vi "Program.vi"() -> ()   [LabVIEW 2018]
panel:
  in  "dados.txt":path
  in  "Error":bool
  in  "Notificacao Rapida":string
  in  "Tab Control":T1(tab)
  in  "DISCREPÂNCIA ACEITA(counts):":u16
  in  "Read-me":bool
  in  "VISUALIZA敲O DE DADOS":bool
  in  "PARAR EXECU敲O":bool
  in  "APAGAR DADOS ANTIGOS":bool
  out "EXECU敲O:":u16
  out "TABELA":string[][](table)
  out "Graph":cluster{"X":dbl[], "Y":dbl[]}[](graph) caption="XY Graph 2"
  in  "Reset":bool
  in  "Enviar Manualmente":bool
  in  "Envio Automático (Horas)":u8
  in  "Senha:":string
  in  "Porta SMTP":string
  in  "SMTP":string
  in  "Assunto:":string
  in  "Para":string[](array[string])
  in  "Email:":string
  in  "Enviar dados para Google Drive":bool
  in  "Enviar notificações por email":bool
  in  "Notificações":string
  in  "counts":dbl[](array[numeric])
  in  "size":i32
  in  "JSONe de Acesso ao Drive":path
  in  "tensao":dbl[](array[numeric])
  # "PAINEL DE CONTROLE"
  # "Gráfico de Counts vs Tensão"
  # "ENVIO DE NOTIFICA钦ES POR EMAIL"
  # "ENVIO AO GOOGLE DRIVE"
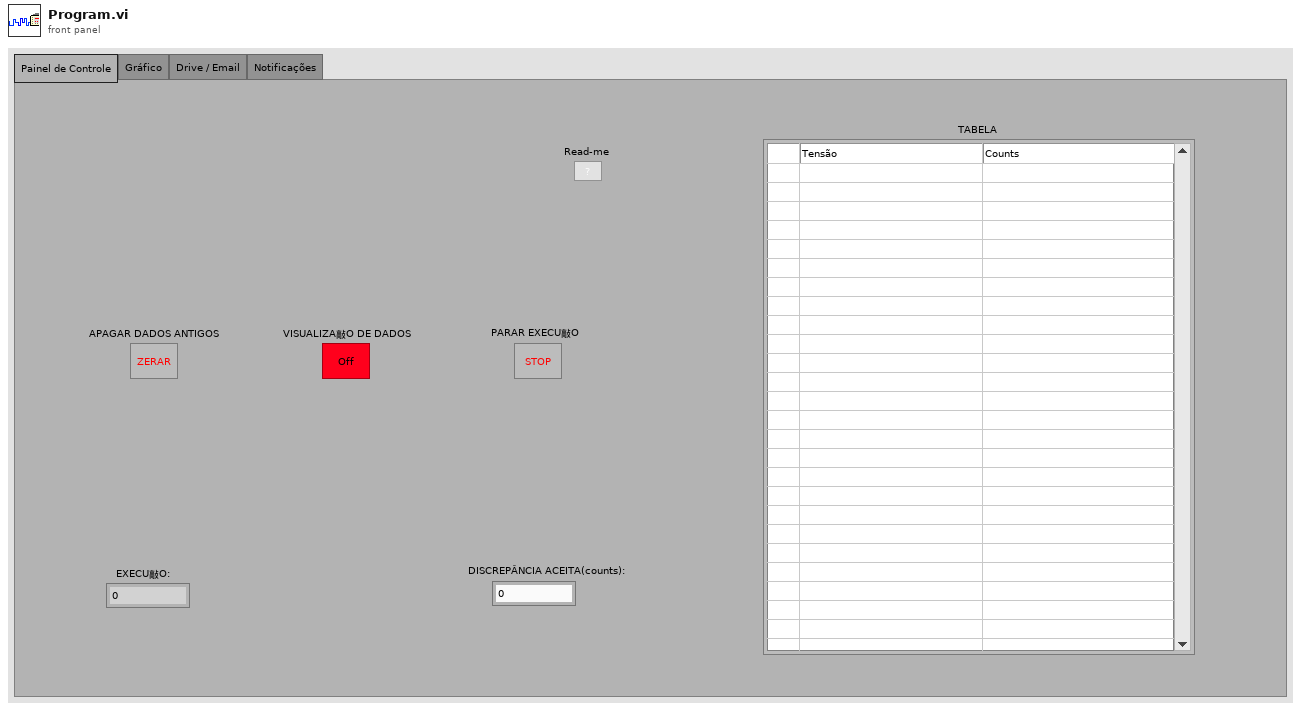
[diagram p1: front panel]
types:
  T1 = enum32{"Painel de Controle", "Gráfico", "Drive / Email", "Notificações"}
  T2 = enum32{"Invalid", "Standard", "Closed", "Hidden", "Minimized", "Maximized"}
  T3 = enum16{"open", "replace", "create", "open or create", "replace or create", "replace or create with confirmation"}
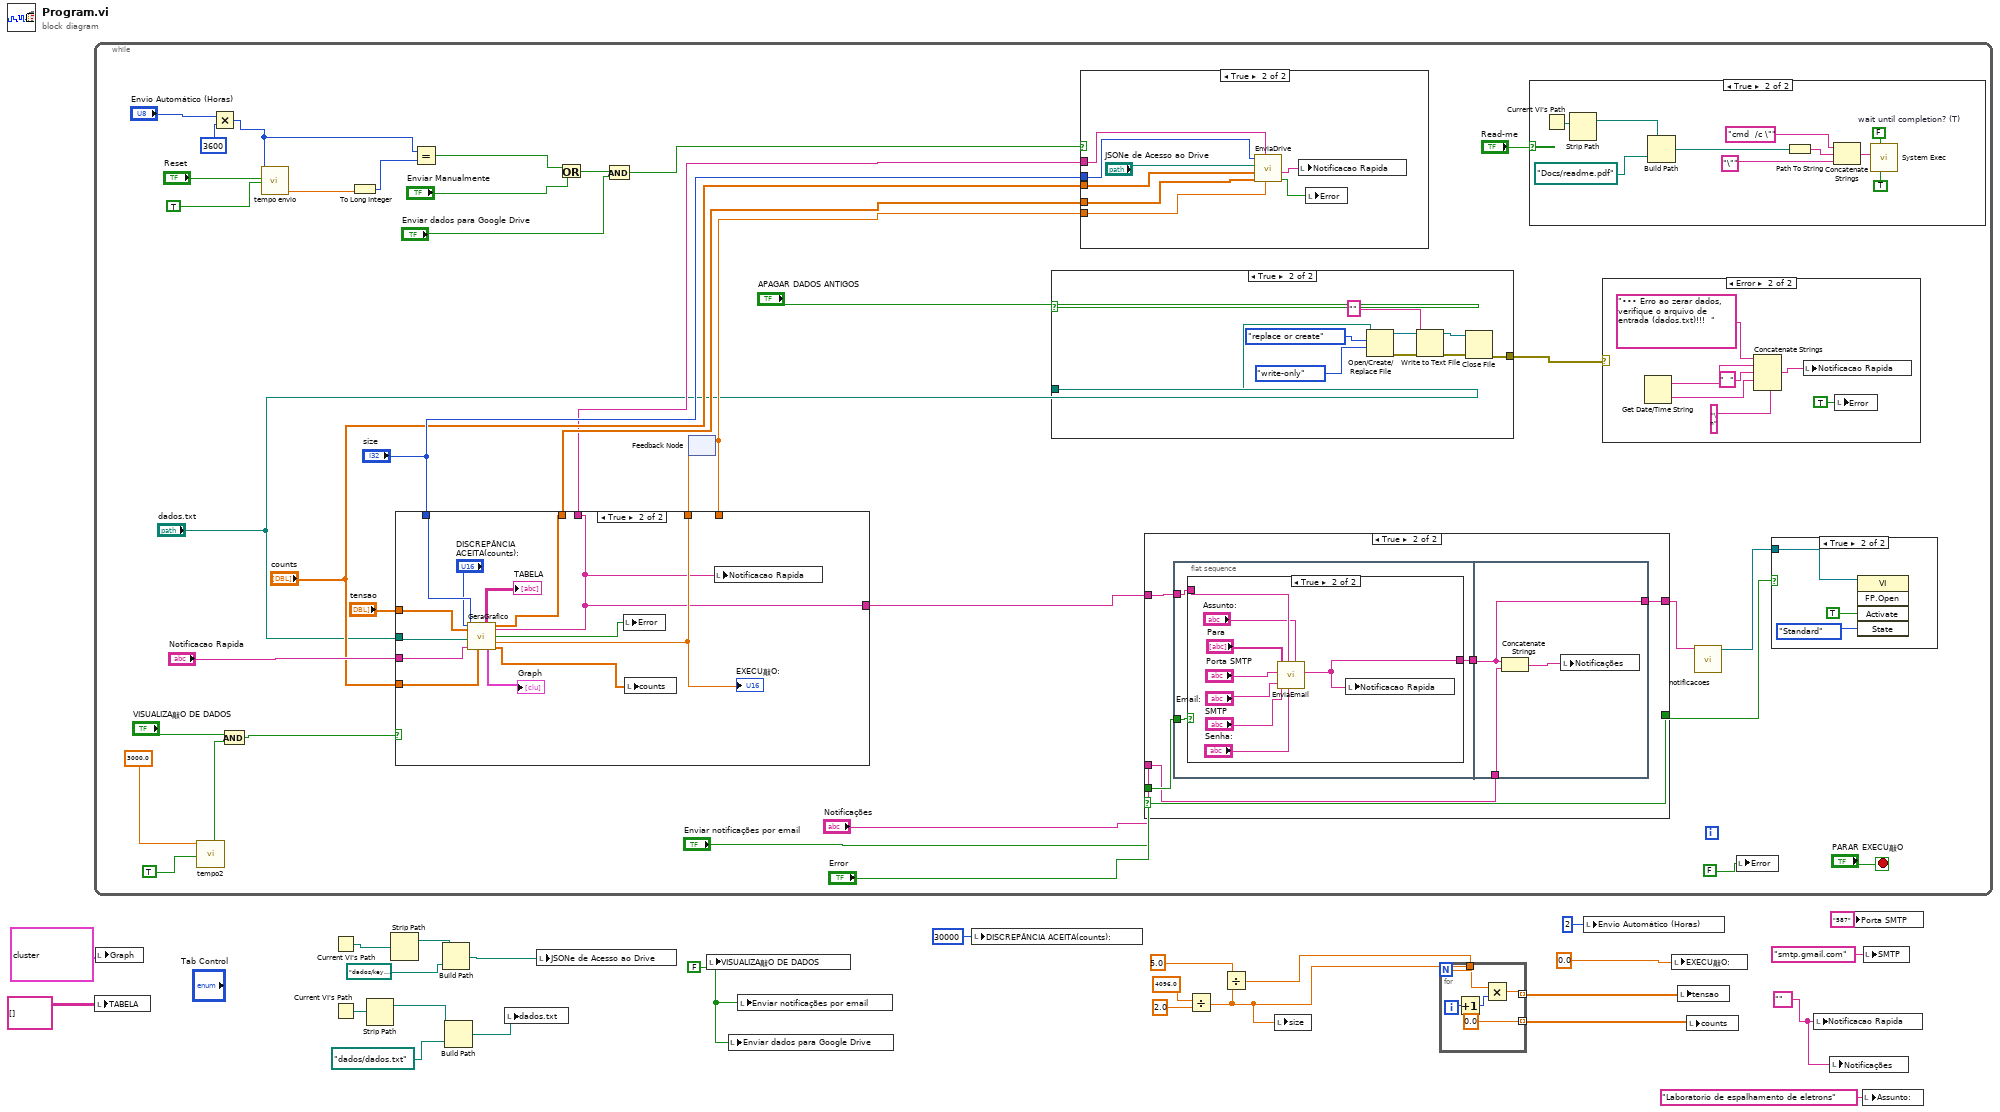
[diagram p0: block diagram]
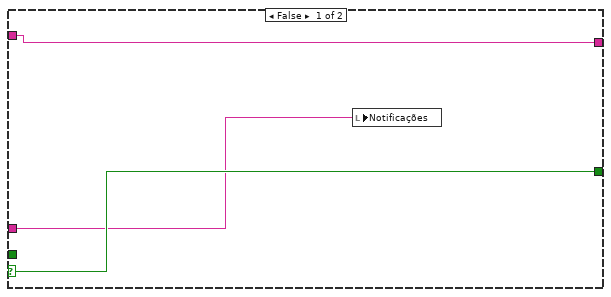
[diagram p4: hidden frame]
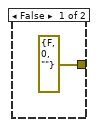
[diagram p7: hidden frame]
diagram:
  w10 = "" ("Notificacoes")
  w2 = FALSE ("Gerar Grafico")
  n1 = while {
    stop <- "PARAR EXECU敲O" stop-if-true
    n2 = call "tempo2"("Time Target (s)"=3000.0, "Auto Reset"=TRUE) -> ("Time has Elapsed"=w54:bool)  [unwired: 10 in, 7 out]
    n3 = Multiply(x="Envio Automático (Horas)", y=u16 3600) -> (x*y=w39:u16)
    n4 = And(x="VISUALIZA敲O DE DADOS", y=w54) -> (x .and. y?=w56:bool)
    n5 = call "tempo envio"("Time Target (s)"=w39, "Reset"="Reset", "Auto Reset"=TRUE) -> ("Elapsed Time (s)"=w63:dbl)  [unwired: 9 in, 7 out]
    n6 = To Long Integer(number=w63) -> (32bit integer=w38:i32)
    n7 = Equal?(x=w39, y=w38) -> (x = y?=w61:bool)
    n8 = Or(x=w61, y="Enviar Manualmente") -> (x .or. y?=w33:bool)
    n9 = And(x=w33, y="Enviar dados para Google Drive") -> (x .and. y?=w32:bool)
    n10 = feedback #1() -> (w46:dbl)  [unwired: 1 in]
    n11 = case shown="True" w56 {
      tunnel: "dados.txt" -> [_ w141]
      tunnel: "size" -> [_ w139]
      tunnel: [w127 w135] -> w49
      tunnel: [w128 w133] -> w47
      tunnel: "Notificacao Rapida" -> [w126 w137]
      tunnel: [w126 w130] -> w37
      tunnel: w46 -> [w128 _]
      tunnel: "tensao" -> [w127 w136]
      tunnel: "counts" -> [_ w131]
      tunnel: [w126 w130] -> w42
      frame False {
      }
      frame True {
        n12 = call "GeraGrafico.vi"("quant"="DISCREPÂNCIA ACEITA(counts):", "Tensao in"=w136, "appended path"=w141, "size"=w139, "notificacao rapida - in"=w137, "counts in"=w131) -> ("notificacao rapida -out"=w130:string, "Tensao out"=w135:dbl[], "Table Control"=→"TABELA":string[][], "error"=w132:bool, "RUN"=w133:dbl, "XY Graph"=→"Graph":cluster{"X":dbl[], "Y":dbl[]}[], "counts out"=w134:dbl[])  [unwired: 3 in]
        "EXECU敲O:" <- w133
        n13 = local write "Error"(w132) -> ()
        n14 = local write "counts"(w134) -> ()
        n15 = local write "Notificacao Rapida"(w130) -> ()
      }
    }
    n16 = feedback-in #1(w47) -> ()
    n17 = case shown="True" "APAGAR DADOS ANTIGOS" {
      tunnel: "dados.txt" -> [_ w112]
      tunnel: [errorcluster {"status"=FALSE, "code"=0, "source"=""} ("error out") w109] -> w36
      frame False {
      }
      frame True {
        n18 = Open/Create/Replace File(file path (use dialog)=w112, operation (0:open)=T3."replace or create", access (0:read/write)=enum16{"read/write", "read-only", "write-only"}."write-only") -> (refnum out=w113:refnum<file>, error out=w116:errorcluster)  [unwired: 3 in, 1 out]
        n19 = Write to Text File(file (use dialog)=w113, text="", error in=w116) -> (refnum out=w111:refnum<file>, error out=w110:errorcluster)  [unwired: 1 in, 1 out]
        n20 = Close File(refnum=w111, error in=w110) -> (error out=w109:errorcluster)  [unwired: 1 out]
      }
    }
    n21 = case shown="True" w32 {
      tunnel: "size" -> [_ w118]
      tunnel: w46 -> [_ w121]
      tunnel: w49 -> [_ w122]
      tunnel: "counts" -> [_ w123]
      tunnel: w42 -> [_ w125]
      frame False {
      }
      frame True {
        n22 = call "EnviaDrive.vi"("run"=w121, "notificacao rapida in"=w125, "tensao in"=w122, "counts in"=w123, "Chave de Acesso ao Drive"="JSONe de Acesso ao Drive", "size"=w118) -> ("Error"=w119:bool, "notificacao rapida out"=w120:string)  [unwired: 4 in]
        n23 = local write "Notificacao Rapida"(w120) -> ()
        n24 = local write "Error"(w119) -> ()
      }
    }
    n25 = case shown="True" "Error" {
      selector: "Error" -> [w83 w89]
      tunnel: [w83 w89] -> w48
      tunnel: w37 -> [w81 w87]
      tunnel: "Notificações" -> [w82 w85]
      tunnel: "Enviar notificações por email" -> [_ w88]
      tunnel: [w81 w84] -> w31
      frame False {
        n26 = local write "Notificações"(w82) -> ()
      }
      frame True {
        n27 = flat-sequence {
          tunnel: w88 -> [w92]
          tunnel: w87 -> [w91]
          tunnel: [w90] -> w86
          tunnel: w86 -> [w102]
          tunnel: w85 -> [w103]
          tunnel: [w102] -> w84
          frame #0 {
            n28 = case shown="True" w92 {
              tunnel: w91 -> [w93 w101]
              tunnel: [w93 w94] -> w90
              frame False {
              }
              frame True {
                n29 = call "EnviaEmail.vi"("subject"="Assunto:", "password"="Senha:", "mensagem"=w101, "SMTP"="SMTP", "username"="Email:", "porta"="Porta SMTP", "Para"="Para") -> ("notificaoes rapidas-out"=w94:string)  [unwired: 4 in]
                n30 = local write "Notificacao Rapida"(w94) -> ()
              }
            }
          }
          frame #1 {
            n31 = Concatenate Strings(w102, w103) -> (w104:string)
            n32 = local write "Notificações"(w104) -> ()
          }
        }
      }
    }
    n33 = case shown="True" "Read-me" {
      frame False {
      }
      frame True {
        w73 = FALSE  # wait until completion? (T)
        n34 = Current VI's Path() -> (path=w66:path)
        n35 = Strip Path(path=w66) -> (stripped path=w67:path)  [unwired: 1 out]
        n36 = Build Path(base path=w67, name or relative path=path "Docs/readme.pdf" ("Path to Secret Client JSON")) -> (appended path=w65:path)
        n37 = Path To String(path=w65) -> (string=w69:string)
        n38 = Concatenate Strings("cmd  /c \"", w69, "\"") -> (w71:string)
        n39 = call <vilib>:"System Exec.vi"("run minimized? (F)"=TRUE, "wait until completion? (T)"=w73, "command line"=w71) -> ()  [unwired: 5 in, 4 out]
      }
    }
    n40 = case shown="Error" w36 {
      frame No Error {
      }
      frame Error {
        n41 = Get Date/Time String() -> (date string=w79:string, time string=w77:string)  [unwired: 3 in]
        n42 = Concatenate Strings("••• Erro ao zerar dados, verifique o arquivo de entrada (dados.txt)!!!  " ("String 3"), w79, "  " ("string"), w77, "\n" ("string")) -> (w75:string)
        n43 = local write "Notificacao Rapida"(w75) -> ()
        n44 = local write "Error"(TRUE ("Error")) -> ()
      }
    }
    n45 = call "notificacoes.vi"("String"=w31) -> ("This VI"=w59:refnum<vi>)  [unwired: 10 out]
    n46 = local write "Error"(FALSE ("Error")) -> ()
    n47 = case shown="True" w48 {
      tunnel: w59 -> [_ w105]
      frame False {
      }
      frame True {
        n48 = invoke class="VI" method="FP.Open"(reference=w105, "Activate"=TRUE ("Activate?"), "State"=T2."Standard") -> ()  [unwired: 2 in, 5 out]
      }
    }
  }
  n49 = local write "TABELA"(string[][] [] ("Table Control")) -> ()
  n50 = local write "Graph"(cluster{"X":dbl[], "Y":dbl[]}[] [{"X"=array[1024 elements], "Y"=array[1024 elements]}] ("Graph")) -> ()
  n51 = Current VI's Path() -> (path=w8:path)
  n52 = Current VI's Path() -> (path=w22:path)
  n53 = Strip Path(path=w8) -> (stripped path=w9:path)  [unwired: 1 out]
  n54 = Strip Path(path=w22) -> (stripped path=w21:path)  [unwired: 1 out]
  n55 = Build Path(base path=w21, name or relative path=path "dados/key.json" ("Path to Secret Client JSON")) -> (appended path=w24:path)
  n56 = Build Path(base path=w9, name or relative path=path "dados/dados.txt" ("Path to Secret Client JSON")) -> (appended path=w6:path)
  n57 = local write "dados.txt"(w6) -> ()
  n58 = local write "JSONe de Acesso ao Drive"(w24) -> ()
  n59 = local write "VISUALIZA敲O DE DADOS"(w2) -> ()
  n60 = local write "Enviar dados para Google Drive"(w2) -> ()
  n61 = local write "Enviar notificações por email"(w2) -> ()
  n62 = local write "DISCREPÂNCIA ACEITA(counts):"(u16 30000 ("DISCREPÂNCIA ACEITA(counts):")) -> ()
  n63 = Divide(x=4096.0 ("y"), y=2.0) -> (x/y=w20:dbl)
  n64 = Divide(x=5.0, y=w20) -> (x/y=w19:dbl)
  n65 = local write "size"(w20) -> ()
  n66 = for {
    N: w20 -> [_]
    tunnel: [w146] -> w18 mode=indexing
    tunnel: w19 -> [w145]
    tunnel: [0.0] -> w14 mode=indexing
    i -> [w143]
    n67 = Increment(x=w143) -> (x+1=w142:i32)
    n68 = Multiply(x=w145, y=w142) -> (x*y=w146:dbl)
  }
  n69 = local write "Envio Automático (Horas)"(u32 2 ("Tempo de Envio (s)")) -> ()
  n70 = local write "EXECU敲O:"(0.0 ("RUN")) -> ()
  n71 = local write "tensao"(w18) -> ()
  n72 = local write "counts"(w14) -> ()
  n73 = local write "Notificacao Rapida"(w10) -> ()
  n74 = local write "Notificações"(w10) -> ()
  n75 = local write "Porta SMTP"("587" ("porta")) -> ()
  n76 = local write "Assunto:"("Laboratorio de espalhamento de eletrons" ("Subject")) -> ()
  n77 = local write "SMTP"("smtp.gmail.com" ("SMTP")) -> ()
